vi "gun_turret_lookup_preset_pos.vi"(11 "Preset Position":T2) -> (3 "Position":T1)   [LabVIEW 2011]
uses:
  gun_preset_pos_t.ctl
  gun_preset_bundle_t.ctl
panel:
  in  "Positions":T1[](array[typedef])=[{"speed"=2200.0, "turret"=0.0, "hood"=75.2, "interval"=1000.0}, {"speed"=2200.0, "turret"=-93.0, "hood"=77.2, "interval"=1000.0}, {"speed"=2200.0, "turret"=100.0, "hood"=77.2, "interval"=1000.0}, {"speed"=2200.0, "turret"=0.0, "hood"=72.0, "interval"=1000.0}, {"speed"=2200.0, "turret"=180.0, "hood"=70.0, "interval"=1000.0}, {"speed"=2200.0, "turret"=90.0, "hood"=96.0, "interval"=1000.0}, {"speed"=2800.0, "turret"=0.0, "hood"=55.0, "interval"=600.0}]
  # "To make it easier on manual user input, these numbers are in terms of pi (1 corresponds to 3.14159)"
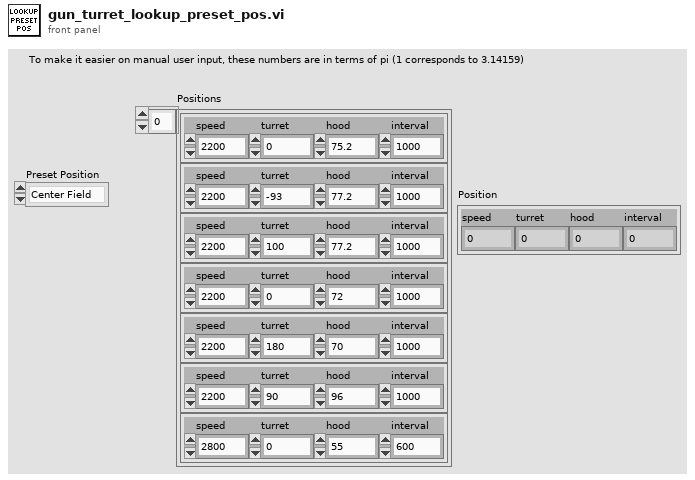
[diagram p1: front panel]
types:
  T1 = typedef "gun_preset_bundle_t.ctl" = cluster{"speed":dbl, "turret":dbl, "hood":dbl, "interval":dbl}
  T2 = typedef "gun_preset_pos_t.ctl" = enum16{"Center Field", "Right Pocket", "Left Pocket", "Align Center", "Align Center Backwards", "Fold Side", "Pass"}
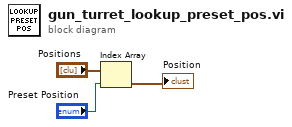
[diagram p0: block diagram]
diagram:
  n1 = Index Array(array="Positions", index="Preset Position") -> (element=→"Position":T1)
